vi "GlobalData.vi"() -> ()   [LabVIEW 2014]
panel:
  out "ChVisible":bool[](array[boolean])
  in  "XAxisName":string[](array[string])
  in  "YAxisName":string[](array[string])
  out "波形グラフref":refnum<vi>
  in  "ヘッダ行":string[][](array[string])
  in  "読捨行":string[][](array[string])
  in  "ChName":string[](array[string])
  in  "ChData":waveform(dbl)[](array[waveform])
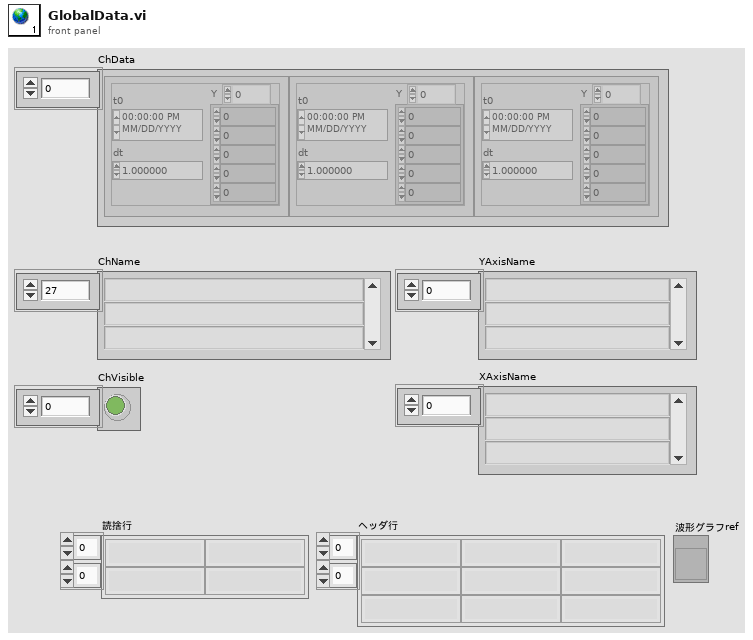
[diagram p1: front panel]
diagram:
